vi "HMI.vi"() -> ()   [LabVIEW 2016]
uses:
  commands.ctl
panel:
  in  "Frequency":dbl(slide) scale=0.0..10.0
  in  "stop":bool
  in  "Command":T1
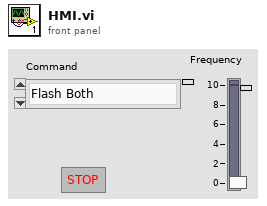
[diagram p1: front panel]
types:
  T1 = typedef "commands.ctl" = enum16{"Flash Both", "Stop All Flash", "Flash FPGA", "Stop FPGA Flash", "Flash RT", "Stop RT Flash"}
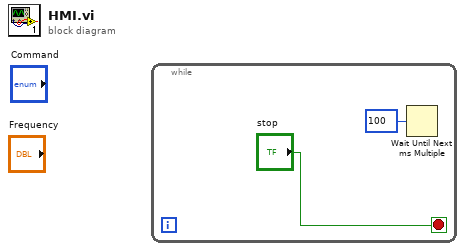
[diagram p0: block diagram]
diagram:
  n1 = while {
    stop <- "stop" stop-if-true
    n2 = Wait Until Next ms Multiple(millisecond multiple=u32 100) -> ()  [unwired: 1 out]
  }
